vi "Add Query.vi"(9 "Value":string, 10 "Name":string, 11 "URI in":refnum<class "URI.lvclass">) -> (3 "URI out":refnum<class "URI.lvclass">)   [LabVIEW 2020, in "URI.lvlib" / "URI.lvclass"]
uses:
  URI.lvclass
  URI.lvclass/URI.ctl
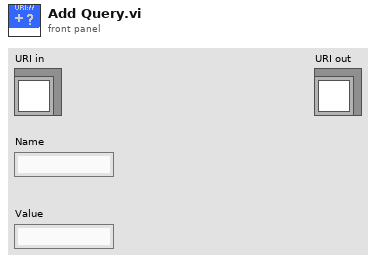
[diagram p1: front panel]
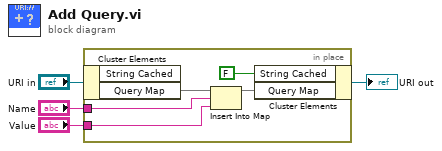
[diagram p0: block diagram]
diagram:
  n1 = in-place {
    in-place-border: "Name" -> [w8]
    in-place-border: "Value" -> [w7]
    n2 = in-place-cluster #1("URI in") -> ("Query Map"=w9:map{string, string})  [unwired: 1 out]
    n3 = Insert Into Map(map in=w9, key=w8, value=w7) -> (map out=w6:map{string, string})  [unwired: 2 out]
    n4 = in-place-cluster #1("String Cached"=FALSE, "Query Map"=w6) -> (→"URI out":refnum<class "URI.lvclass">)
  }
